vi "Winch v6.vi"() -> ()   [LabVIEW 2013]
uses:
  Globals/Data for Dashboard.vi
  <vilib>/Rock Robotics/WPI/Joystick/WPI_JoystickGetSetRefNum.vi
  Robot Global Data.vi
  Globals/Useful Values.vi
  Globals/Homes.vi
  <vilib>/addons/control/pid/pid.llb/PID (DBL).vi
  <vilib>/Utility/file.llb/Write To Spreadsheet File (DBL).vi
  <vilib>/addons/control/pid/NI_PID_pid.lvlib
panel:
  in  "Winch Out Amoun":dbl=3.95 format="%#_13g"
  out "Winch Armed?":bool
  out "Winch Power":bool
  in  "PID gains":T1={"proportional gain (Kc)"=2.75, "integral time (Ti, min)"=0.0, "derivative time (Td, min)"=0.0} {"derivative time (Td, min)" format="%.3f"; "integral time (Ti, min)" format="%.3f"; "proportional gain (Kc)" format="%.3f"}
  # "PULLBACK SPEED NEEDS\nTO BE NEGATIVE OR ELSE"
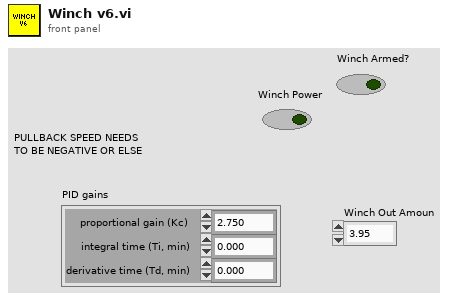
[diagram p1: front panel]
types:
  T1 = cluster{"proportional gain (Kc)":dbl, "integral time (Ti, min)":dbl, "derivative time (Td, min)":dbl}
  T2 = typedef "WPI_DigitalInputDevRef.ctl" = cluster{"DevStatus":errorcluster, "DIO Channel":T3, "Digital Module":T4}
  T3 = typedef "FPGA_DIOChannel.ctl" = enum8{"DIO 1", "DIO 2", "DIO 3", "DIO 4", "DIO 5", "DIO 6", "DIO 7", "DIO 8", "DIO 9", "DIO 10", "DIO 11", "DIO 12", "DIO 13", "DIO 14", "Invalid"}
  T4 = typedef "FPGA_TypedefDigitalModule.ctl" = enum16{"Digital Module 1", "Digital Module 2"}
  T5 = typedef "WPI_JoystickDevRef.ctl" = cluster{"Device":T6}
  T6 = typedef "WPI_JoystickDeviceEnum.ctl" = enum16{"USB 1", "USB 2", "USB 3", "USB 4", "Kinect 1", "Kinect 2"}
  T7 = typedef "WPI_MotorControlDeviceRef.ctl" = cluster{"DeviceStatus":errorcluster, "Type":enum16{"PWM", "CAN"}, "PWM":cluster{"Digital Module":T4, "PWM Channel":T8, "DeadBand":T9}, "CAN":cluster{"Device Number":u8, "Control Mode":T10, "Semaphore":T11, "Max Vout":dbl}, "Invert":bool, "TransformRef":T12, "InvTransformRef":T12}
  T8 = typedef "FPGA_DIOPWMChannel.ctl" = enum8{"PWM 1", "PWM 2", "PWM 3", "PWM 4", "PWM 5", "PWM 6", "PWM 7", "PWM 8", "PWM 9", "PWM 10", "Invalid"}
  T9 = typedef "WPI_PWMDeadband.ctl" = cluster{"Name":string, "maxPositivePwm":i32, "minPositivePwm":i32, "centerPwm":i32, "maxNegativePwm":i32, "minNegativePwm":i32, "angularRange":u16}
  T10 = typedef "WPI_CANJaguar_ControlMode.ctl" = enum8{"Percent VBus", "Current", "Speed", "Position", "Voltage"}
  T11 = typedef "Semaphore RefNum" = refnum<k1>
  T12 = typedef "WPI_PWMTransform_ConPane.ctl" = refnum<vi>
  T13 = typedef "WPI_AnalogChannelDevRef.ctl" = cluster{"DevStatus":errorcluster, "Analog Module":T14, "Analog Channel":T15}
  T14 = typedef "FPGA_TypedefAnalogModule.ctl" = enum16{"Analog Module 1", "Analog Module 2"}
  T15 = typedef "FPGA_AIChannel.ctl" = enum8{"AI 1", "AI 2", "AI 3", "AI 4", "AI 5", "AI 6", "AI 7", "AI 8", "Invalid"}
  T16 = typedef "WPI_DriverStationRobotMode2.ctl" = enum16{"Autonomous Disabled", "Autonomous Enabled", "Teleop Disabled", "Teleop Enabled", "Timeout", "Finish", "Test Disabled", "Test Enabled"}
  T17 = typedef "WPI_JoystickButtonState.ctl" = cluster{"Button 1":bool, "Button 2":bool, "Button 3":bool, "Button 4":bool, "Button 5":bool, "Button 6":bool, "Button 7":bool, "Button 8":bool, "Button 9":bool, "Button 10":bool, "Button 11":bool, "Button 12":bool}
  T18 = cluster{"axis 1 (x)":dbl, "axis 2 (y)":dbl, "axis 3 (throttle)":dbl, "axis 4":dbl, "axis 5":dbl, "axis 6":dbl}
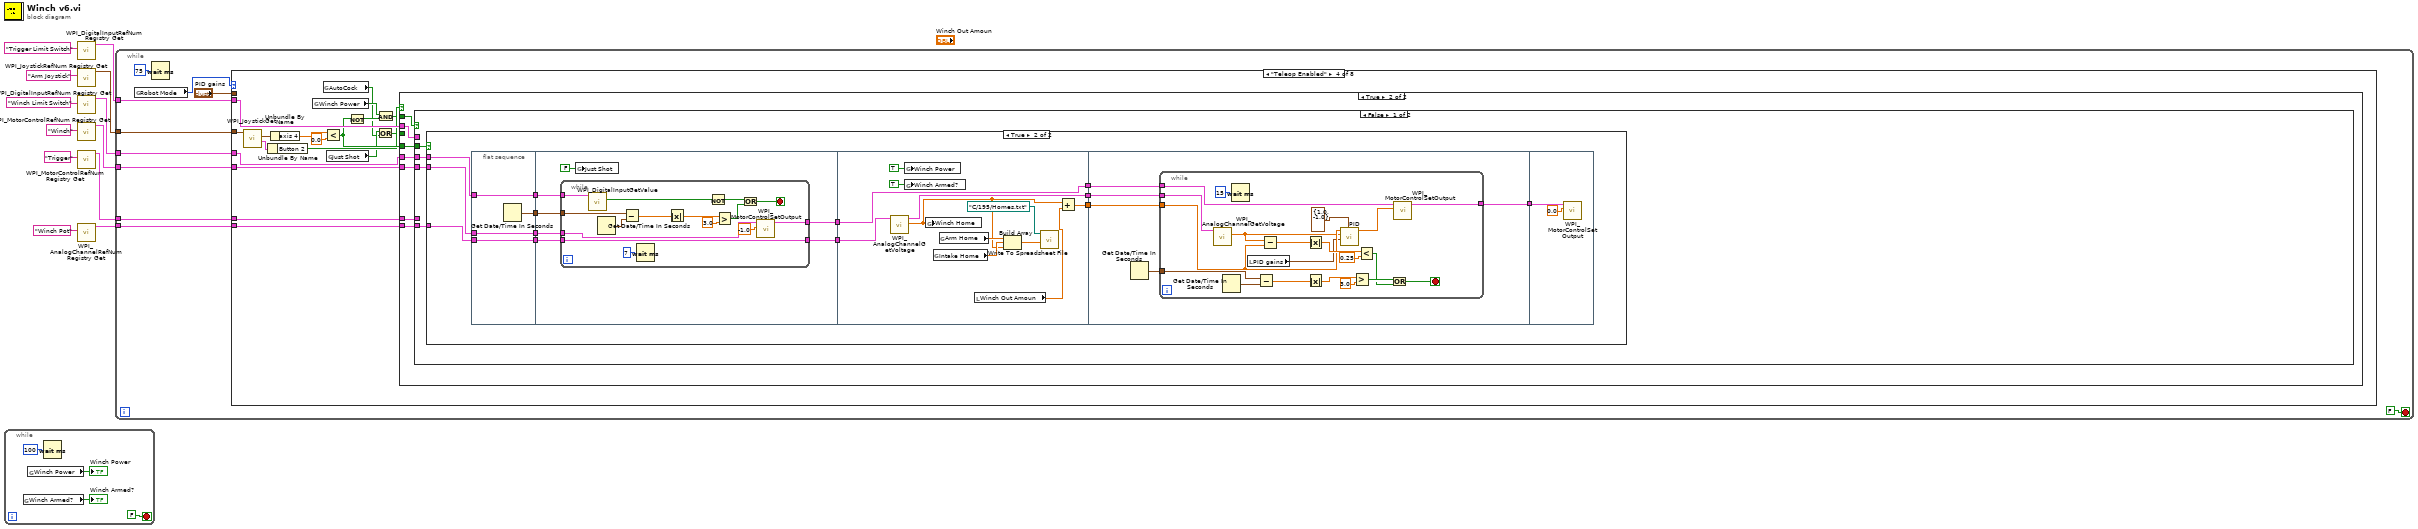
[diagram p0: block diagram]
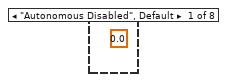
[diagram p2: hidden frame]
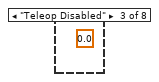
[diagram p4: hidden frame]
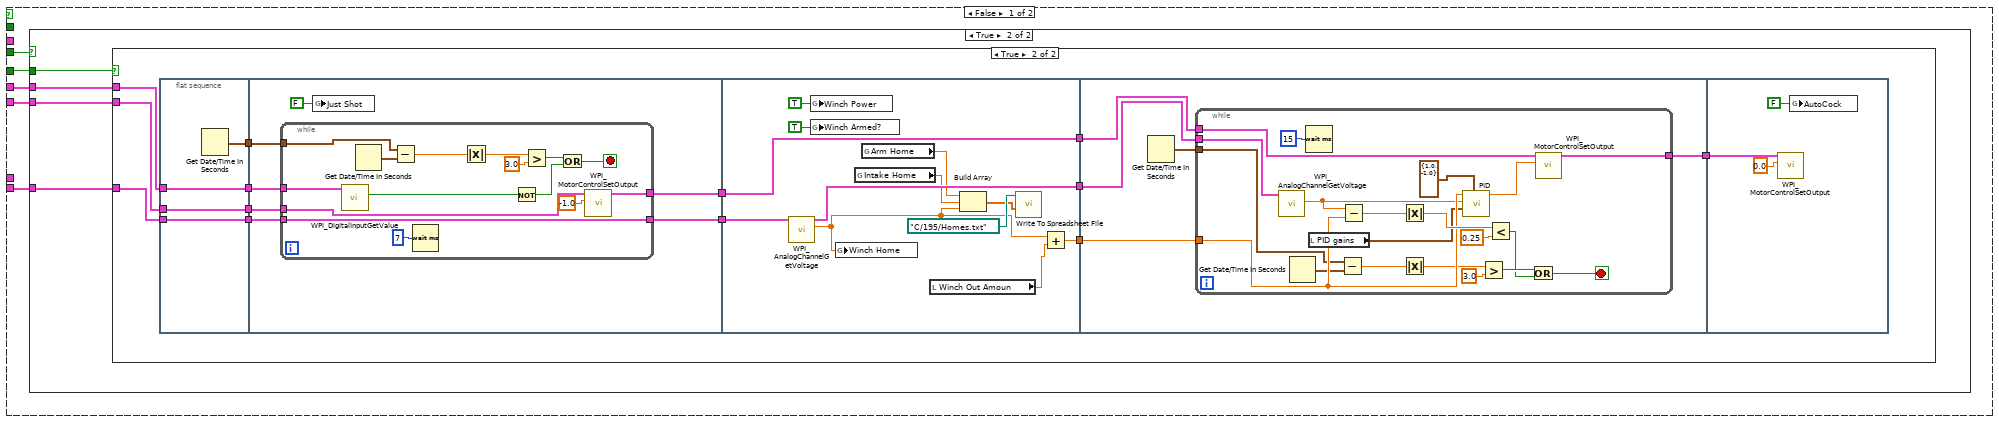
[diagram p5: hidden frame]
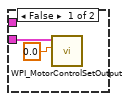
[diagram p6: hidden frame]
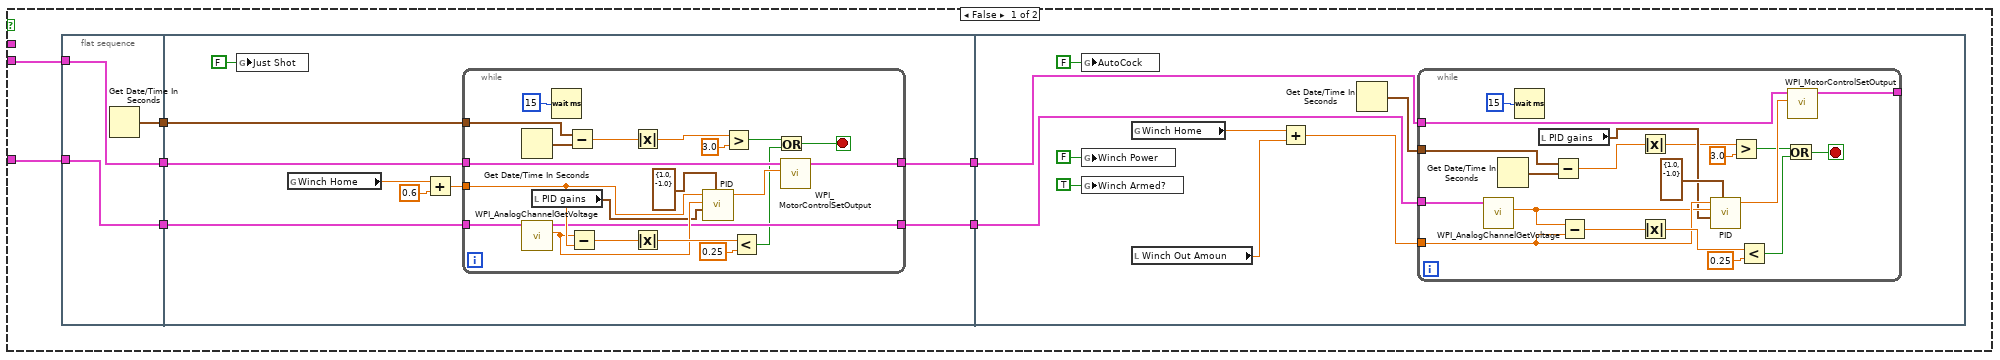
[diagram p7: hidden frame]
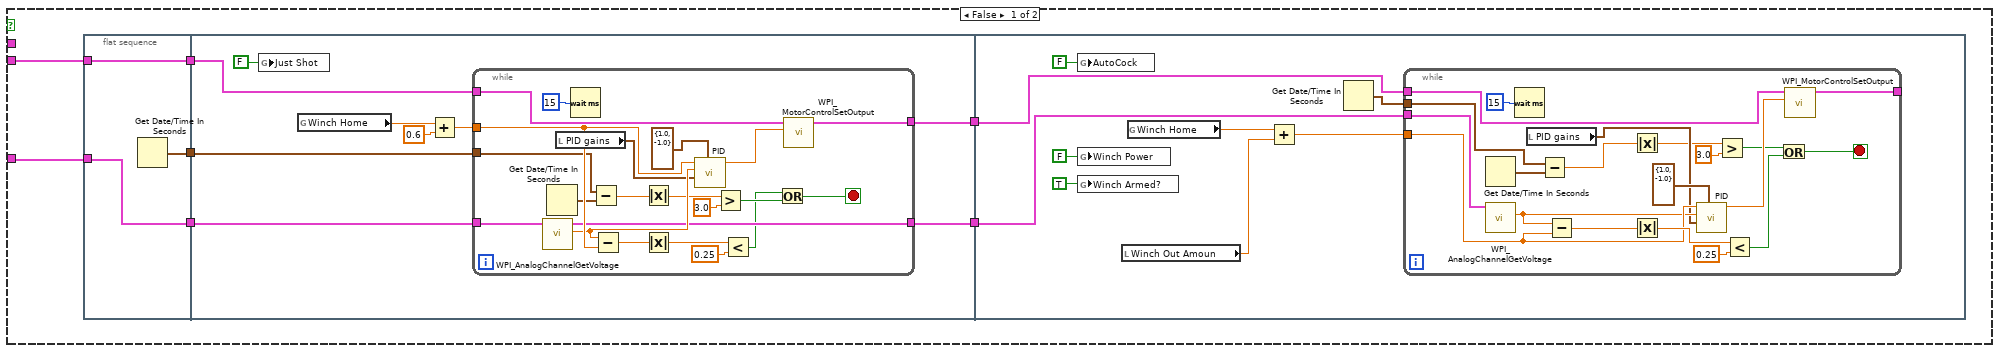
[diagram p8: hidden frame]
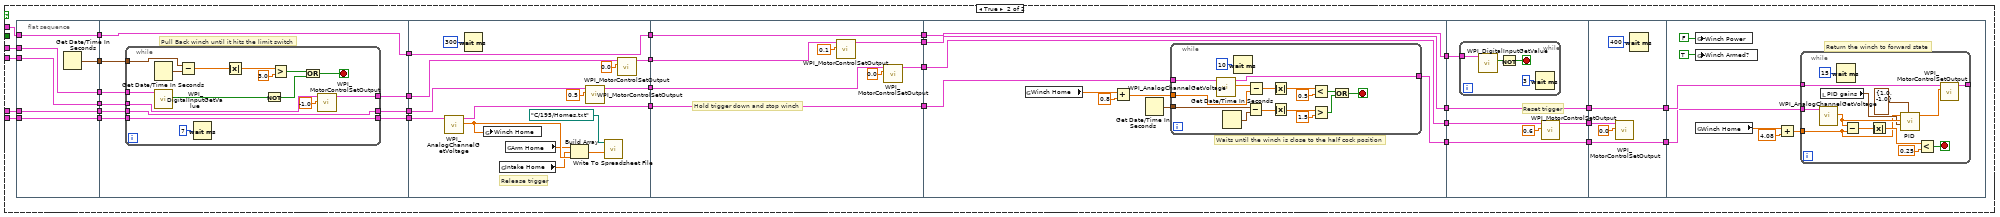
[diagram p9: hidden frame]
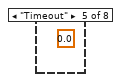
[diagram p10: hidden frame]
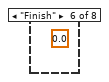
[diagram p11: hidden frame]
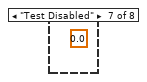
[diagram p12: hidden frame]
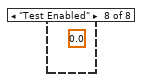
[diagram p13: hidden frame]
diagram:
  n1 = while {
    stop <- FALSE stop-if-true
    n2 = global read "Data for Dashboard.vi" "Winch Armed?"() -> (→"Winch Armed?":bool)
    n3 = global read "Data for Dashboard.vi" "Winch Power"() -> (→"Winch Power":bool)
    n4 = Wait (ms)(milliseconds to wait=u32 100) -> ()  [unwired: 1 out]
  }
  n5 = call <vilib>:"WPI_DigitalInputRefNum Registry Get.vi"("refnum name"="Trigger Limit Switch") -> ("DigitalInputDevRef"=w1:T2)  [unwired: 9 in, 1 out]
  n6 = call <vilib>:"WPI_JoystickRefNum Registry Get.vi"("refnum name"="Arm Joystick") -> ("JoystickDevRef"=w7:T5)  [unwired: 9 in, 1 out]
  n7 = call <vilib>:"WPI_DigitalInputRefNum Registry Get.vi"("refnum name"="Winch Limit Switch") -> ("DigitalInputDevRef"=w6:T2)  [unwired: 9 in, 1 out]
  n8 = call <vilib>:"WPI_MotorControlRefNum Registry Get.vi"("refnum name"="Winch") -> ("MotorControlDevRef"=w9:T7)  [unwired: 9 in, 1 out]
  n9 = call <vilib>:"WPI_MotorControlRefNum Registry Get.vi"("refnum name"="Trigger") -> ("MotorControlDevRef"=w3:T7)  [unwired: 9 in, 1 out]
  n10 = call <vilib>:"WPI_AnalogChannelRefNum Registry Get.vi"("refnum name"="Winch Pot") -> ("AIDeviceRef"=w12:T13)  [unwired: 9 in, 1 out]
  n11 = while {
    tunnel: w12 -> [w18]
    tunnel: w9 -> [w17]
    tunnel: w7 -> [w22]
    tunnel: w6 -> [w20]
    tunnel: w3 -> [w21]
    tunnel: w1 -> [w19]
    stop <- FALSE stop-if-true
    n12 = global read "Robot Global Data.vi" "Robot Mode"() -> (w24:T16)
    n13 = Wait (ms)(milliseconds to wait=u32 75) -> ()  [unwired: 1 out]
    n14 = case shown="\"Teleop Enabled\"" w24 {
      tunnel: w17 -> [_ _ _ w41 _ _ _ _]
      tunnel: "PID gains" -> [_ _ _ _ _ _ _ _]
      tunnel: w22 -> [_ _ _ w44 _ _ _ _]
      tunnel: w20 -> [_ _ _ w42 _ _ _ _]
      tunnel: w18 -> [_ _ _ w40 _ _ _ _]
      tunnel: w21 -> [_ _ _ w39 _ _ _ _]
      tunnel: w19 -> [_ _ _ w38 _ _ _ _]
      frame "Autonomous Disabled", Default {
        (unwired) 0.0 ("Motor Output")
      }
      frame "Autonomous Enabled" {
      }
      frame "Teleop Disabled" {
        (unwired) 0.0 ("Motor Output")
      }
      frame "Teleop Enabled" {
        n15 = call <vilib>:"WPI_JoystickGet.vi"("JoystickDevRef"=w44) -> ("Buttons"=w43:T17, "Axes"=w36:T18)  [unwired: 4 in, 1 out]
        n16 = Unbundle By Name(w43) -> ("Button 2"=w31:bool)
        n17 = Unbundle By Name(w36) -> ("axis 4"=w35:dbl)
        n18 = global read "Data for Dashboard.vi" "Winch Power"() -> (w37:bool)
        n19 = global read "Useful Values.vi" "AutoCock"() -> (w28:bool)
        n20 = Less?(x=w35, y=0.0) -> (x < y?=w33:bool)
        n21 = global read "Useful Values.vi" "Just Shot"() -> (w29:bool)
        n22 = Not(x=w33) -> (.not. x?=w32:bool)
        n23 = Or(x=w29, y=w28) -> (x .or. y?=w27:bool)
        n24 = And(x=w37, y=w32) -> (x .and. y?=w30:bool)
        n25 = case shown="True" w31 {
          tunnel: w42 -> [w47 w208]
          tunnel: w41 -> [w49 w210]
          tunnel: w40 -> [w46 w209]
          tunnel: w39 -> [_ w207]
          tunnel: w38 -> [_ w206]
          tunnel: w30 -> [_ w205]
          tunnel: w33 -> [w45 w204]
          tunnel: w27 -> [w48 _]
          frame False {
            n26 = case shown="True" w48 {
              tunnel: w49 -> [w51 w54]
              tunnel: w47 -> [_ w55]
              tunnel: w46 -> [_ w53]
              tunnel: w45 -> [_ w52]
              frame False {
                n27 = call <vilib>:"WPI_MotorControlSetOutput.vi"("Output"=0.0, "MotorControlDevRef"=w51) -> ()  [unwired: 7 in, 3 out]
              }
              frame True {
                n28 = case shown="True" w52 {
                  tunnel: w54 -> [w61 w131]
                  tunnel: w53 -> [w62 w130]
                  tunnel: w55 -> [_ w129]
                  frame False {
                    n29 = flat-sequence {
                      tunnel: w62 -> [w64]
                      tunnel: w61 -> [w65]
                      tunnel: [w65] -> w58
                      tunnel: [w64] -> w57
                      tunnel: [w63] -> w56
                      tunnel: [w69] -> w60
                      tunnel: [w68] -> w59
                      tunnel: w58 -> [w74]
                      tunnel: w57 -> [w73]
                      tunnel: w56 -> [w66]
                      tunnel: w60 -> [w104]
                      tunnel: w59 -> [w103]
                      frame #0 {
                        n30 = Get Date/Time In Seconds() -> (seconds since 1Jan1904=w63:timestamp)
                      }
                      frame #1 {
                        n31 = global write "Useful Values.vi" "Just Shot"(FALSE ("Just Shot")) -> ()
                        n32 = global read "Homes.vi" "Winch Home"() -> (w72:dbl)
                        n33 = Add(x=w72, y=0.6) -> (x+y=w70:dbl)
                        n34 = while {
                          tunnel: w74 -> [w95]
                          tunnel: w70 -> [w89]
                          tunnel: w73 -> [w91]
                          tunnel: [w87] -> w69
                          tunnel: [w83] -> w68
                          tunnel: w66 -> [w78]
                          stop <- w76 stop-if-true
                          n35 = Get Date/Time In Seconds() -> (seconds since 1Jan1904=w79:timestamp)
                          n36 = call <vilib>:"WPI_AnalogChannelGetVoltage.vi"("AIDeviceRef"=w91) -> ("Voltage"=w88:dbl, "AIDeviceRef"=w83:T13)  [unwired: 8 in, 1 out]
                          n37 = local read "PID gains"() -> (w86:T1)
                          n38 = Wait (ms)(milliseconds to wait=u32 15) -> ()  [unwired: 1 out]
                          n39 = Subtract(x=w78, y=w79) -> (x-y=w80:dbl)
                          n40 = Subtract(x=w88, y=w89) -> (x-y=w94:dbl)
                          n41 = Absolute Value(x=w80) -> (abs(x)=w81:dbl)
                          n42 = Absolute Value(x=w94) -> (abs(x)=w93:dbl)
                          n43 = call-poly <vilib>:"PID.vi"("output range"=cluster{"output high":dbl, "output low":dbl} {"output high"=1.0, "output low"=-1.0}, "PID gains"=w86, "process variable"=w88, "setpoint"=w89) -> ("output"=w84:dbl)  [unwired: 6 in, 1 out]
                          n44 = Greater?(x=w81, y=3.0) -> (0:w77:bool)
                          n45 = Less?(x=w93, y=0.25) -> (x < y?=w75:bool)
                          n46 = Or(x=w77, y=w75) -> (x .or. y?=w76:bool)
                          n47 = call <vilib>:"WPI_MotorControlSetOutput.vi"("Output"=w84, "MotorControlDevRef"=w95) -> ("MotorControlDevRef"=w87:T7)  [unwired: 7 in, 2 out]
                        }
                      }
                      frame #2 {
                        n48 = global write "Useful Values.vi" "AutoCock"(FALSE ("AutoCock")) -> ()
                        n49 = global write "Data for Dashboard.vi" "Winch Power"(FALSE ("Loaded")) -> ()
                        n50 = global write "Data for Dashboard.vi" "Winch Armed?"(TRUE ("Loaded")) -> ()
                        n51 = global read "Homes.vi" "Winch Home"() -> (w102:dbl)
                        n52 = local read "Winch Out Amoun"() -> (w96:dbl)
                        n53 = Add(x=w102, y=w96) -> (x+y=w101:dbl)
                        n54 = Get Date/Time In Seconds() -> (seconds since 1Jan1904=w97:timestamp)
                        n55 = while {
                          tunnel: w104 -> [w124]
                          tunnel: w101 -> [w118]
                          tunnel: w103 -> [w120]
                          tunnel: [w116] -> _
                          tunnel: w97 -> [w107]
                          stop <- w105 stop-if-true
                          n56 = call <vilib>:"WPI_AnalogChannelGetVoltage.vi"("AIDeviceRef"=w120) -> ("Voltage"=w117:dbl)  [unwired: 8 in, 2 out]
                          n57 = Get Date/Time In Seconds() -> (seconds since 1Jan1904=w111:timestamp)
                          n58 = Wait (ms)(milliseconds to wait=u32 15) -> ()  [unwired: 1 out]
                          n59 = local read "PID gains"() -> (w115:T1)
                          n60 = Subtract(x=w107, y=w111) -> (x-y=w110:dbl)
                          n61 = Subtract(x=w117, y=w118) -> (x-y=w123:dbl)
                          n62 = Absolute Value(x=w110) -> (abs(x)=w109:dbl)
                          n63 = Absolute Value(x=w123) -> (abs(x)=w122:dbl)
                          n64 = call-poly <vilib>:"PID.vi"("output range"=cluster{"output high":dbl, "output low":dbl} {"output high"=1.0, "output low"=-1.0}, "PID gains"=w115, "process variable"=w117, "setpoint"=w118) -> ("output"=w113:dbl)  [unwired: 6 in, 1 out]
                          n65 = Greater?(x=w109, y=3.0) -> (0:w112:bool)
                          n66 = Less?(x=w122, y=0.25) -> (x < y?=w106:bool)
                          n67 = Or(x=w112, y=w106) -> (x .or. y?=w105:bool)
                          n68 = call <vilib>:"WPI_MotorControlSetOutput.vi"("Output"=w113, "MotorControlDevRef"=w124) -> ("MotorControlDevRef"=w116:T7)  [unwired: 7 in, 2 out]
                        }
                      }
                    }
                  }
                  frame True {
                    n69 = flat-sequence {
                      tunnel: w130 -> [w139]
                      tunnel: w131 -> [w140]
                      tunnel: w129 -> [w141]
                      tunnel: [w141] -> w128
                      tunnel: [w140] -> w127
                      tunnel: [w139] -> w126
                      tunnel: [w138] -> w125
                      tunnel: [w146] -> w137
                      tunnel: [w143] -> w136
                      tunnel: w128 -> [w148]
                      tunnel: w127 -> [w147]
                      tunnel: w126 -> [w144]
                      tunnel: w125 -> [w142]
                      tunnel: w137 -> [w175]
                      tunnel: [w175] -> w135
                      tunnel: [w174] -> w134
                      tunnel: w136 -> [w173]
                      tunnel: [w172] -> w133
                      tunnel: w135 -> [w180]
                      tunnel: w134 -> [w178]
                      tunnel: [w177] -> w132
                      tunnel: w133 -> [w179]
                      tunnel: w132 -> [w203]
                      frame #0 {
                        n70 = Get Date/Time In Seconds() -> (seconds since 1Jan1904=w138:timestamp)
                      }
                      frame #1 {
                        n71 = while {
                          tunnel: w148 -> [w163]
                          tunnel: w147 -> [w159]
                          tunnel: [w158] -> w146
                          tunnel: w144 -> [w157]
                          tunnel: [w157] -> w143
                          tunnel: w142 -> [w156]
                          stop <- w149 stop-if-true
                          n72 = call <vilib>:"WPI_DigitalInputGetValue.vi"("DigitalInputDevRef"=w163) -> ("Value"=w162:bool)  [unwired: 8 in, 2 out]
                          n73 = Get Date/Time In Seconds() -> (seconds since 1Jan1904=w155:timestamp)
                          n74 = Subtract(x=w156, y=w155) -> (x-y=w154:dbl)
                          n75 = Wait (ms)(milliseconds to wait=u32 7) -> ()  [unwired: 1 out]
                          n76 = Absolute Value(x=w154) -> (abs(x)=w153:dbl)
                          n77 = Not(x=w162) -> (.not. x?=w150:bool)
                          n78 = Greater?(x=w153, y=3.0) -> (0:w151:bool)
                          n79 = Or(x=w151, y=w150) -> (x .or. y?=w149:bool)
                          n80 = call <vilib>:"WPI_MotorControlSetOutput.vi"("Output"=-1.0 ("Pullback Speed"), "MotorControlDevRef"=w159) -> ("MotorControlDevRef"=w158:T7)  [unwired: 7 in, 2 out]
                        }
                        n81 = global write "Useful Values.vi" "Just Shot"(FALSE ("Just Shot")) -> ()
                      }
                      frame #2 {
                        n82 = call <vilib>:"WPI_AnalogChannelGetVoltage.vi"("AIDeviceRef"=w173) -> ("Voltage"=w167:dbl, "AIDeviceRef"=w174:T13)  [unwired: 8 in, 1 out]
                        n83 = global write "Data for Dashboard.vi" "Winch Power"(TRUE ("Loaded")) -> ()
                        n84 = global write "Data for Dashboard.vi" "Winch Armed?"(TRUE ("Loaded")) -> ()
                        n85 = global write "Homes.vi" "Winch Home"(w167) -> ()
                        n86 = global read "Homes.vi" "Intake Home"() -> (w168:dbl)
                        n87 = global read "Homes.vi" "Arm Home"() -> (w170:dbl)
                        n88 = local read "Winch Out Amoun"() -> (w164:dbl)
                        n89 = Build Array(w170, w168, w167) -> (w169:dbl[])
                        n90 = call-poly <vilib>:"Write To Spreadsheet File.vi"("1D data"=w169, "file path (dialog if empty)"=path "C:/195/Homes.txt") -> ()  [unwired: 6 in, 1 out]
                        n91 = Add(x=w167, y=w164) -> (x+y=w172:dbl)
                      }
                      frame #3 {
                        n92 = Get Date/Time In Seconds() -> (seconds since 1Jan1904=w176:timestamp)
                        n93 = while {
                          tunnel: w180 -> [w200]
                          tunnel: w179 -> [w194]
                          tunnel: w178 -> [w196]
                          tunnel: [w192] -> w177
                          tunnel: w176 -> [w183]
                          stop <- w181 stop-if-true
                          n94 = call <vilib>:"WPI_AnalogChannelGetVoltage.vi"("AIDeviceRef"=w196) -> ("Voltage"=w193:dbl)  [unwired: 8 in, 2 out]
                          n95 = Get Date/Time In Seconds() -> (seconds since 1Jan1904=w187:timestamp)
                          n96 = Wait (ms)(milliseconds to wait=u32 15) -> ()  [unwired: 1 out]
                          n97 = local read "PID gains"() -> (w191:T1)
                          n98 = Subtract(x=w183, y=w187) -> (x-y=w186:dbl)
                          n99 = Subtract(x=w193, y=w194) -> (x-y=w199:dbl)
                          n100 = Absolute Value(x=w199) -> (abs(x)=w198:dbl)
                          n101 = Absolute Value(x=w186) -> (abs(x)=w185:dbl)
                          n102 = call-poly <vilib>:"PID.vi"("output range"=cluster{"output high":dbl, "output low":dbl} {"output high"=1.0, "output low"=-1.0}, "PID gains"=w191, "process variable"=w193, "setpoint"=w194) -> ("output"=w189:dbl)  [unwired: 6 in, 1 out]
                          n103 = Greater?(x=w185, y=3.0) -> (0:w188:bool)
                          n104 = Less?(x=w198, y=0.25) -> (x < y?=w182:bool)
                          n105 = Or(x=w188, y=w182) -> (x .or. y?=w181:bool)
                          n106 = call <vilib>:"WPI_MotorControlSetOutput.vi"("Output"=w189, "MotorControlDevRef"=w200) -> ("MotorControlDevRef"=w192:T7)  [unwired: 7 in, 2 out]
                        }
                      }
                      frame #4 {
                        n107 = call <vilib>:"WPI_MotorControlSetOutput.vi"("Output"=0.0, "MotorControlDevRef"=w203) -> ()  [unwired: 7 in, 3 out]
                        n108 = global write "Useful Values.vi" "AutoCock"(FALSE ("AutoCock")) -> ()
                      }
                    }
                  }
                }
              }
            }
          }
          frame True {
            n109 = case shown="False" w205 {
              tunnel: w210 -> [w213 w372]
              tunnel: w209 -> [w212 w371]
              tunnel: w208 -> [w211 w370]
              tunnel: w207 -> [_ w369]
              tunnel: w206 -> [_ w368]
              tunnel: w204 -> [w214 _]
              frame False {
                n110 = case shown="True" w214 {
                  tunnel: w213 -> [w220 w290]
                  tunnel: w212 -> [w221 w289]
                  tunnel: w211 -> [_ w288]
                  frame False {
                    n111 = flat-sequence {
                      tunnel: w221 -> [w223]
                      tunnel: w220 -> [w224]
                      tunnel: [w224] -> w217
                      tunnel: [w223] -> w216
                      tunnel: [w222] -> w215
                      tunnel: [w228] -> w219
                      tunnel: [w227] -> w218
                      tunnel: w217 -> [w233]
                      tunnel: w216 -> [w232]
                      tunnel: w215 -> [w225]
                      tunnel: w219 -> [w263]
                      tunnel: w218 -> [w262]
                      frame #0 {
                        n112 = Get Date/Time In Seconds() -> (seconds since 1Jan1904=w222:timestamp)
                      }
                      frame #1 {
                        n113 = global write "Useful Values.vi" "Just Shot"(FALSE ("Just Shot")) -> ()
                        n114 = global read "Homes.vi" "Winch Home"() -> (w231:dbl)
                        n115 = Add(x=w231, y=0.6) -> (x+y=w229:dbl)
                        n116 = while {
                          tunnel: w233 -> [w254]
                          tunnel: w229 -> [w248]
                          tunnel: w232 -> [w250]
                          tunnel: [w246] -> w228
                          tunnel: [w242] -> w227
                          tunnel: w225 -> [w237]
                          stop <- w234 stop-if-true
                          n117 = call <vilib>:"WPI_AnalogChannelGetVoltage.vi"("AIDeviceRef"=w250) -> ("Voltage"=w247:dbl, "AIDeviceRef"=w242:T13)  [unwired: 8 in, 1 out]
                          n118 = Get Date/Time In Seconds() -> (seconds since 1Jan1904=w238:timestamp)
                          n119 = local read "PID gains"() -> (w245:T1)
                          n120 = Wait (ms)(milliseconds to wait=u32 15) -> ()  [unwired: 1 out]
                          n121 = Subtract(x=w237, y=w238) -> (x-y=w239:dbl)
                          n122 = Subtract(x=w247, y=w248) -> (x-y=w253:dbl)
                          n123 = Absolute Value(x=w239) -> (abs(x)=w240:dbl)
                          n124 = Absolute Value(x=w253) -> (abs(x)=w252:dbl)
                          n125 = call-poly <vilib>:"PID.vi"("output range"=cluster{"output high":dbl, "output low":dbl} {"output high"=1.0, "output low"=-1.0}, "PID gains"=w245, "process variable"=w247, "setpoint"=w248) -> ("output"=w243:dbl)  [unwired: 6 in, 1 out]
                          n126 = Greater?(x=w240, y=3.0) -> (0:w236:bool)
                          n127 = Less?(x=w252, y=0.25) -> (x < y?=w235:bool)
                          n128 = Or(x=w235, y=w236) -> (x .or. y?=w234:bool)
                          n129 = call <vilib>:"WPI_MotorControlSetOutput.vi"("Output"=w243, "MotorControlDevRef"=w254) -> ("MotorControlDevRef"=w246:T7)  [unwired: 7 in, 2 out]
                        }
                      }
                      frame #2 {
                        n130 = global write "Useful Values.vi" "AutoCock"(FALSE ("AutoCock")) -> ()
                        n131 = global write "Data for Dashboard.vi" "Winch Power"(FALSE ("Loaded")) -> ()
                        n132 = global write "Data for Dashboard.vi" "Winch Armed?"(TRUE ("Loaded")) -> ()
                        n133 = local read "Winch Out Amoun"() -> (w255:dbl)
                        n134 = global read "Homes.vi" "Winch Home"() -> (w261:dbl)
                        n135 = Add(x=w261, y=w255) -> (x+y=w260:dbl)
                        n136 = Get Date/Time In Seconds() -> (seconds since 1Jan1904=w256:timestamp)
                        n137 = while {
                          tunnel: w263 -> [w283]
                          tunnel: w260 -> [w277]
                          tunnel: w262 -> [w279]
                          tunnel: [w275] -> _
                          tunnel: w256 -> [w264]
                          stop <- w266 stop-if-true
                          n138 = Get Date/Time In Seconds() -> (seconds since 1Jan1904=w268:timestamp)
                          n139 = call <vilib>:"WPI_AnalogChannelGetVoltage.vi"("AIDeviceRef"=w279) -> ("Voltage"=w276:dbl)  [unwired: 8 in, 2 out]
                          n140 = Wait (ms)(milliseconds to wait=u32 15) -> ()  [unwired: 1 out]
                          n141 = local read "PID gains"() -> (w274:T1)
                          n142 = Subtract(x=w264, y=w268) -> (x-y=w269:dbl)
                          n143 = Subtract(x=w276, y=w277) -> (x-y=w282:dbl)
                          n144 = Absolute Value(x=w269) -> (abs(x)=w270:dbl)
                          n145 = Absolute Value(x=w282) -> (abs(x)=w281:dbl)
                          n146 = call-poly <vilib>:"PID.vi"("output range"=cluster{"output high":dbl, "output low":dbl} {"output high"=1.0, "output low"=-1.0}, "PID gains"=w274, "process variable"=w276, "setpoint"=w277) -> ("output"=w272:dbl)  [unwired: 6 in, 1 out]
                          n147 = Greater?(x=w270, y=3.0) -> (0:w267:bool)
                          n148 = Less?(x=w281, y=0.25) -> (x < y?=w265:bool)
                          n149 = Or(x=w267, y=w265) -> (x .or. y?=w266:bool)
                          n150 = call <vilib>:"WPI_MotorControlSetOutput.vi"("Output"=w272, "MotorControlDevRef"=w283) -> ("MotorControlDevRef"=w275:T7)  [unwired: 7 in, 2 out]
                        }
                      }
                    }
                  }
                  frame True {
                    n151 = flat-sequence {
                      tunnel: w289 -> [w298]
                      tunnel: w290 -> [w299]
                      tunnel: w288 -> [w300]
                      tunnel: [w300] -> w287
                      tunnel: [w299] -> w286
                      tunnel: [w298] -> w285
                      tunnel: [w297] -> w284
                      tunnel: [w305] -> w296
                      tunnel: [w302] -> w295
                      tunnel: w287 -> [w307]
                      tunnel: w286 -> [w306]
                      tunnel: w285 -> [w303]
                      tunnel: w284 -> [w301]
                      tunnel: w296 -> [w334]
                      tunnel: [w334] -> w294
                      tunnel: [w333] -> w293
                      tunnel: w295 -> [w332]
                      tunnel: [w331] -> w292
                      tunnel: w294 -> [w339]
                      tunnel: w293 -> [w337]
                      tunnel: [w336] -> w291
                      tunnel: w292 -> [w338]
                      tunnel: w291 -> [w361]
                      frame #0 {
                        n152 = Get Date/Time In Seconds() -> (seconds since 1Jan1904=w297:timestamp)
                      }
                      frame #1 {
                        n153 = while {
                          tunnel: w307 -> [w322]
                          tunnel: w306 -> [w318]
                          tunnel: [w317] -> w305
                          tunnel: w303 -> [w314]
                          tunnel: [w314] -> w302
                          tunnel: w301 -> [w309]
                          stop <- w316 stop-if-true
                          n154 = call <vilib>:"WPI_DigitalInputGetValue.vi"("DigitalInputDevRef"=w322) -> ("Value"=w321:bool)  [unwired: 8 in, 2 out]
                          n155 = Get Date/Time In Seconds() -> (seconds since 1Jan1904=w313:timestamp)
                          n156 = Subtract(x=w309, y=w313) -> (x-y=w312:dbl)
                          n157 = Wait (ms)(milliseconds to wait=u32 7) -> ()  [unwired: 1 out]
                          n158 = Absolute Value(x=w312) -> (abs(x)=w311:dbl)
                          n159 = Not(x=w321) -> (.not. x?=w315:bool)
                          n160 = Greater?(x=w311, y=3.0) -> (0:w308:bool)
                          n161 = Or(x=w315, y=w308) -> (x .or. y?=w316:bool)
                          n162 = call <vilib>:"WPI_MotorControlSetOutput.vi"("Output"=-1.0 ("Pullback Speed"), "MotorControlDevRef"=w318) -> ("MotorControlDevRef"=w317:T7)  [unwired: 7 in, 2 out]
                        }
                        n163 = global write "Useful Values.vi" "Just Shot"(FALSE ("Just Shot")) -> ()
                      }
                      frame #2 {
                        n164 = call <vilib>:"WPI_AnalogChannelGetVoltage.vi"("AIDeviceRef"=w332) -> ("Voltage"=w326:dbl, "AIDeviceRef"=w333:T13)  [unwired: 8 in, 1 out]
                        n165 = global write "Data for Dashboard.vi" "Winch Power"(TRUE ("Loaded")) -> ()
                        n166 = global write "Data for Dashboard.vi" "Winch Armed?"(TRUE ("Loaded")) -> ()
                        n167 = global write "Homes.vi" "Winch Home"(w326) -> ()
                        n168 = global read "Homes.vi" "Intake Home"() -> (w327:dbl)
                        n169 = global read "Homes.vi" "Arm Home"() -> (w329:dbl)
                        n170 = local read "Winch Out Amoun"() -> (w323:dbl)
                        n171 = Build Array(w329, w327, w326) -> (w328:dbl[])
                        n172 = call-poly <vilib>:"Write To Spreadsheet File.vi"("1D data"=w328, "file path (dialog if empty)"=path "C:/195/Homes.txt") -> ()  [unwired: 6 in, 1 out]
                        n173 = Add(x=w326, y=w323) -> (x+y=w331:dbl)
                      }
                      frame #3 {
                        n174 = Get Date/Time In Seconds() -> (seconds since 1Jan1904=w335:timestamp)
                        n175 = while {
                          tunnel: w339 -> [w359]
                          tunnel: w338 -> [w353]
                          tunnel: w337 -> [w355]
                          tunnel: [w351] -> w336
                          tunnel: w335 -> [w340]
                          stop <- w341 stop-if-true
                          n176 = call <vilib>:"WPI_AnalogChannelGetVoltage.vi"("AIDeviceRef"=w355) -> ("Voltage"=w352:dbl)  [unwired: 8 in, 2 out]
                          n177 = Get Date/Time In Seconds() -> (seconds since 1Jan1904=w344:timestamp)
                          n178 = Wait (ms)(milliseconds to wait=u32 15) -> ()  [unwired: 1 out]
                          n179 = local read "PID gains"() -> (w350:T1)
                          n180 = Subtract(x=w340, y=w344) -> (x-y=w345:dbl)
                          n181 = Subtract(x=w352, y=w353) -> (x-y=w358:dbl)
                          n182 = Absolute Value(x=w358) -> (abs(x)=w357:dbl)
                          n183 = Absolute Value(x=w345) -> (abs(x)=w346:dbl)
                          n184 = call-poly <vilib>:"PID.vi"("output range"=cluster{"output high":dbl, "output low":dbl} {"output high"=1.0, "output low"=-1.0}, "PID gains"=w350, "process variable"=w352, "setpoint"=w353) -> ("output"=w348:dbl)  [unwired: 6 in, 1 out]
                          n185 = Greater?(x=w346, y=3.0) -> (0:w343:bool)
                          n186 = Less?(x=w357, y=0.25) -> (x < y?=w342:bool)
                          n187 = Or(x=w343, y=w342) -> (x .or. y?=w341:bool)
                          n188 = call <vilib>:"WPI_MotorControlSetOutput.vi"("Output"=w348, "MotorControlDevRef"=w359) -> ("MotorControlDevRef"=w351:T7)  [unwired: 7 in, 2 out]
                        }
                      }
                      frame #4 {
                        n189 = call <vilib>:"WPI_MotorControlSetOutput.vi"("Output"=0.0, "MotorControlDevRef"=w361) -> ()  [unwired: 7 in, 3 out]
                      }
                    }
                  }
                }
              }
              frame True {
                n190 = flat-sequence {
                  tunnel: w368 -> [w395]
                  tunnel: w369 -> [w396]
                  tunnel: w370 -> [w397]
                  tunnel: w371 -> [w398]
                  tunnel: w372 -> [w399]
                  tunnel: [w399] -> w367
                  tunnel: [w398] -> w366
                  tunnel: [w397] -> w365
                  tunnel: [w396] -> w364
                  tunnel: [w395] -> w363
                  tunnel: [w394] -> w362
                  tunnel: [w405] -> w393
                  tunnel: [w403] -> w392
                  tunnel: [w402] -> w391
                  tunnel: [w401] -> w390
                  tunnel: w367 -> [w408]
                  tunnel: w366 -> [w407]
                  tunnel: w365 -> [w406]
                  tunnel: w364 -> [w404]
                  tunnel: w363 -> [w401]
                  tunnel: w362 -> [w400]
                  tunnel: w393 -> [w439]
                  tunnel: [w436] -> w389
                  tunnel: [w425] -> w388
                  tunnel: w392 -> [w427]
                  tunnel: w391 -> [w429]
                  tunnel: [w428] -> w387
                  tunnel: [w435] -> w386
                  tunnel: w390 -> [w435]
                  tunnel: w389 -> [w447]
                  tunnel: w388 -> [w444]
                  tunnel: w387 -> [w445]
                  tunnel: [w445] -> w385
                  tunnel: [w443] -> w384
                  tunnel: [w441] -> w383
                  tunnel: w386 -> [w441]
                  tunnel: [w440] -> w382
                  tunnel: w385 -> [w455]
                  tunnel: w384 -> [w456]
                  tunnel: [w456] -> w381
                  tunnel: [w451] -> w380
                  tunnel: w383 -> [w451]
                  tunnel: w382 -> [w450]
                  tunnel: [w450] -> w379
                  tunnel: [w449] -> w378
                  tunnel: w381 -> [w478]
                  tunnel: [w478] -> w377
                  tunnel: w380 -> [w477]
                  tunnel: w379 -> [w475]
                  tunnel: [w474] -> w376
                  tunnel: w378 -> [w473]
                  tunnel: [w473] -> w375
                  tunnel: w377 -> [w487]
                  tunnel: [w487] -> w374
                  tunnel: w376 -> [w483]
                  tunnel: w375 -> [w486]
                  tunnel: [w486] -> w373
                  tunnel: w374 -> [w494]
                  tunnel: w373 -> [w493]
                  frame #0 {
                    n191 = Get Date/Time In Seconds() -> (seconds since 1Jan1904=w394:timestamp)
                  }
                  frame #1 {
                    # "Pull Back winch until it hits the limit switch"
                    n192 = while {
                      tunnel: [w421] -> w403
                      tunnel: w408 -> [w420]
                      tunnel: w407 -> [w417]
                      tunnel: w406 -> [w419]
                      tunnel: [w418] -> w405
                      tunnel: w404 -> [w418]
                      tunnel: [w417] -> w402
                      tunnel: w400 -> [w412]
                      stop <- w410 stop-if-true
                      n193 = Get Date/Time In Seconds() -> (seconds since 1Jan1904=w413:timestamp)
                      n194 = call <vilib>:"WPI_DigitalInputGetValue.vi"("DigitalInputDevRef"=w419) -> ("Value"=w424:bool)  [unwired: 8 in, 2 out]
                      n195 = Subtract(x=w412, y=w413) -> (x-y=w414:dbl)
                      n196 = Wait (ms)(milliseconds to wait=u32 7) -> ()  [unwired: 1 out]
                      n197 = Absolute Value(x=w414) -> (abs(x)=w415:dbl)
                      n198 = Not(x=w424) -> (.not. x?=w411:bool)
                      n199 = Greater?(x=w415, y=3.0) -> (0:w409:bool)
                      n200 = Or(x=w409, y=w411) -> (x .or. y?=w410:bool)
                      n201 = call <vilib>:"WPI_MotorControlSetOutput.vi"("Output"=-1.0 ("Pullback Speed"), "MotorControlDevRef"=w420) -> ("MotorControlDevRef"=w421:T7)  [unwired: 7 in, 2 out]
                    }
                  }
                  frame #2 {
                    # "Release trigger"
                    n202 = call <vilib>:"WPI_AnalogChannelGetVoltage.vi"("AIDeviceRef"=w429) -> ("Voltage"=w434:dbl, "AIDeviceRef"=w428:T13)  [unwired: 8 in, 1 out]
                    n203 = Wait (ms)(milliseconds to wait=u32 300) -> ()  [unwired: 1 out]
                    n204 = global write "Homes.vi" "Winch Home"(w434) -> ()
                    n205 = global read "Homes.vi" "Intake Home"() -> (w433:dbl)
                    n206 = global read "Homes.vi" "Arm Home"() -> (w431:dbl)
                    n207 = Build Array(w431, w433, w434) -> (w432:dbl[])
                    n208 = call <vilib>:"WPI_MotorControlSetOutput.vi"("Output"=0.5, "MotorControlDevRef"=w439) -> ("MotorControlDevRef"=w436:T7)  [unwired: 7 in, 2 out]
                    n209 = call-poly <vilib>:"Write To Spreadsheet File.vi"("1D data"=w432, "file path (dialog if empty)"=path "C:/195/Homes.txt") -> ()  [unwired: 6 in, 1 out]
                    n210 = call <vilib>:"WPI_MotorControlSetOutput.vi"("Output"=0.0, "MotorControlDevRef"=w427) -> ("MotorControlDevRef"=w425:T7)  [unwired: 7 in, 2 out]
                  }
                  frame #3 {
                    # "Hold trigger down and stop winch"
                    n211 = call <vilib>:"WPI_MotorControlSetOutput.vi"("Output"=0.1, "MotorControlDevRef"=w444) -> ("MotorControlDevRef"=w443:T7)  [unwired: 7 in, 2 out]
                    n212 = call <vilib>:"WPI_MotorControlSetOutput.vi"("Output"=0.0, "MotorControlDevRef"=w447) -> ("MotorControlDevRef"=w440:T7)  [unwired: 7 in, 2 out]
                  }
                  frame #4 {
                    # "Waits until the winch is close to the half cock position"
                    n213 = global read "Homes.vi" "Winch Home"() -> (w454:dbl)
                    n214 = Add(x=w454, y=0.8) -> (x+y=w452:dbl)
                    n215 = Get Date/Time In Seconds() -> (seconds since 1Jan1904=w448:timestamp)
                    n216 = while {
                      tunnel: w455 -> [w472]
                      tunnel: w452 -> [w466]
                      tunnel: [w465] -> w449
                      tunnel: w448 -> [w457]
                      stop <- w458 stop-if-true
                      n217 = call <vilib>:"WPI_AnalogChannelGetVoltage.vi"("AIDeviceRef"=w472) -> ("Voltage"=w471:dbl, "AIDeviceRef"=w465:T13)  [unwired: 8 in, 1 out]
                      n218 = Get Date/Time In Seconds() -> (seconds since 1Jan1904=w463:timestamp)
                      n219 = Wait (ms)(milliseconds to wait=u32 10) -> ()  [unwired: 1 out]
                      n220 = Subtract(x=w457, y=w463) -> (x-y=w462:dbl)
                      n221 = Subtract(x=w471, y=w466) -> (x-y=w470:dbl)
                      n222 = Absolute Value(x=w470) -> (abs(x)=w469:dbl)
                      n223 = Absolute Value(x=w462) -> (abs(x)=w461:dbl)
                      n224 = Less?(x=w469, y=0.5) -> (x < y?=w459:bool)
                      n225 = Greater?(x=w461, y=1.5) -> (0:w464:bool)
                      n226 = Or(x=w459, y=w464) -> (x .or. y?=w458:bool)
                    }
                  }
                  frame #5 {
                    # "Reset trigger"
                    n227 = while {
                      tunnel: w477 -> [w482]
                      stop <- w480 stop-if-true
                      n228 = call <vilib>:"WPI_DigitalInputGetValue.vi"("DigitalInputDevRef"=w482) -> ("Value"=w481:bool)  [unwired: 8 in, 2 out]
                      n229 = Not(x=w481) -> (.not. x?=w480:bool)
                      n230 = Wait (ms)(milliseconds to wait=u32 3) -> ()  [unwired: 1 out]
                    }
                    n231 = call <vilib>:"WPI_MotorControlSetOutput.vi"("Output"=0.6, "MotorControlDevRef"=w475) -> ("MotorControlDevRef"=w474:T7)  [unwired: 7 in, 2 out]
                  }
                  frame #6 {
                    n232 = call <vilib>:"WPI_MotorControlSetOutput.vi"("Output"=0.0, "MotorControlDevRef"=w483) -> ()  [unwired: 7 in, 3 out]
                    n233 = Wait (ms)(milliseconds to wait=u32 400) -> ()  [unwired: 1 out]
                  }
                  frame #7 {
                    # "Return the winch to forward state"
                    n234 = global write "Data for Dashboard.vi" "Winch Power"(FALSE ("Loaded")) -> ()
                    n235 = global write "Data for Dashboard.vi" "Winch Armed?"(TRUE ("Loaded")) -> ()
                    n236 = global read "Homes.vi" "Winch Home"() -> (w492:dbl)
                    n237 = Add(x=w492, y=4.08) -> (x+y=w490:dbl)
                    n238 = while {
                      tunnel: w494 -> [w507]
                      tunnel: [w500] -> _
                      tunnel: w493 -> [w496]
                      tunnel: w490 -> [w495]
                      stop <- w504 stop-if-true
                      n239 = call <vilib>:"WPI_AnalogChannelGetVoltage.vi"("AIDeviceRef"=w496) -> ("Voltage"=w501:dbl)  [unwired: 8 in, 2 out]
                      n240 = local read "PID gains"() -> (w499:T1)
                      n241 = Wait (ms)(milliseconds to wait=u32 15) -> ()  [unwired: 1 out]
                      n242 = Subtract(x=w501, y=w495) -> (x-y=w506:dbl)
                      n243 = Absolute Value(x=w506) -> (abs(x)=w505:dbl)
                      n244 = call-poly <vilib>:"PID.vi"("output range"=cluster{"output high":dbl, "output low":dbl} {"output high"=1.0, "output low"=-1.0}, "PID gains"=w499, "process variable"=w501, "setpoint"=w495) -> ("output"=w497:dbl)  [unwired: 6 in, 1 out]
                      n245 = Less?(x=w505, y=0.25) -> (x < y?=w504:bool)
                      n246 = call <vilib>:"WPI_MotorControlSetOutput.vi"("Output"=w497, "MotorControlDevRef"=w507) -> ("MotorControlDevRef"=w500:T7)  [unwired: 7 in, 2 out]
                    }
                  }
                }
              }
            }
          }
        }
      }
      frame "Timeout" {
        (unwired) 0.0 ("Motor Output")
      }
      frame "Finish" {
        (unwired) 0.0 ("Motor Output")
      }
      frame "Test Disabled" {
        (unwired) 0.0 ("Motor Output")
      }
      frame "Test Enabled" {
        (unwired) 0.0 ("Motor Output")
      }
    }
  }
